vi "Get Gyro Sim Data Path.vi"(2 "APDM Context":T1={"APDM Context ID"=0, "Gyro Mode"="", "Log Data"=FALSE, "Log File"=refnum, "Gyro Record Log"=refnum, "Gyro CMD Log"=refnum, "L Opal SN"=0, "R Opal SN"=0, "Access Point ID"=0, "Left Gyro Sim Data"=path "C:/Users/jfalesi/Desktop/CP FES Walking Code/Original/Ahad Vi/CP Code/Offline data/TD_7_Raw_R.txt", "Right Gyro Sim Data"=path "C:/Users/jfalesi/Desktop/CP FES Walking Code/Original/Ahad Vi/CP Code/Offline data/TD_7_Raw_R.txt", "Sampling Rate"=0.0, "Gyro Sim Time Array"=[], "Missed Gyro Count"=0.0}, 3 "Left or Right":T2) -> (1 "Gyro Sim Data Path":path)   [LabVIEW 2019]
uses:
  Archive/CP_FES_Walking_w_stim_on_off.llb/Left_Right_Control.ctl
  Controls/APDM Context Cluster.ctl
panel:
  out "L or R":string
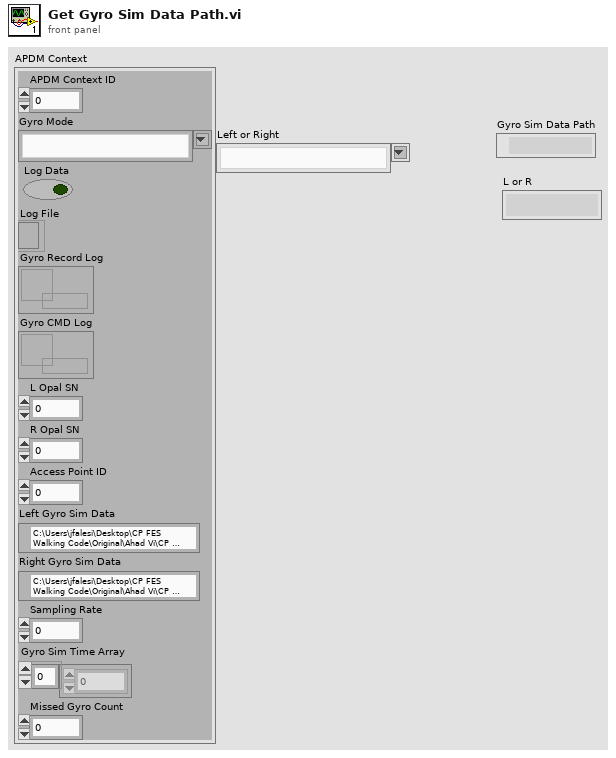
[diagram p1: front panel]
types:
  T1 = typedef "APDM Context Cluster.ctl" = cluster{"APDM Context ID":u32, "Gyro Mode":string, "Log Data":bool, "Log File":refnum<file>, "Gyro Record Log":refnum<queue>, "Gyro CMD Log":refnum<queue>, "L Opal SN":u32, "R Opal SN":u32, "Access Point ID":u32, "Left Gyro Sim Data":path, "Right Gyro Sim Data":path, "Sampling Rate":dbl, "Gyro Sim Time Array":dbl[], "Missed Gyro Count":dbl}
  T2 = typedef "Left_Right_Control.ctl" = string
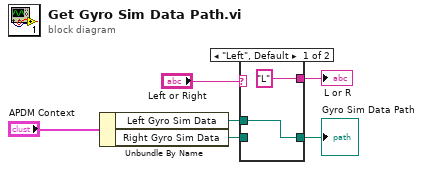
[diagram p0: block diagram]
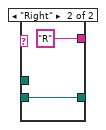
[diagram p2: hidden frame]
diagram:
  n1 = Unbundle By Name("APDM Context") -> ("Left Gyro Sim Data"=w4:path, "Right Gyro Sim Data"=w3:path)
  n2 = case shown="\"Left\", Default" "Left or Right" {
    tunnel: w4 -> [w8 _]
    tunnel: w3 -> [_ w10]
    tunnel: [w8 w10] -> w1
    tunnel: ["L" "R"] -> w5
    frame "Left", Default {
    }
    frame "Right" {
    }
  }
  "L or R" <- w5
  "Gyro Sim Data Path" <- w1
